vi "TEST_InputDevice.vi"() -> ()   [LabVIEW 2021, in "InputDevice.lvlib"]
uses:
  InputDevice.lvlib
  Joystick/Joystick.lvclass
  Keyboard/Keyboard.lvclass
  Mouse/Mouse.lvclass
  <vilib>/ErrorRing/Error Ring.xnode
  InputDevice.lvclass
  5e27b7e4-08c8-4db0-82d1-7d7273c4f812.vi
  <vilib>/Utility/miscctls.llb/LVPoint32TypeDef.ctl
panel:
  out "mouse info":T1(array[cluster])
  out "key info":T2(array[cluster])
  out "joystick info":T3(array[cluster])
  out "Joystick B Info Button 1":bool
  out "Joystick Axis Events":T4
  out "Joy Direction Event":T5
  out "Keys Pressed":T6(array[ring])
  out "Button Info Event":T7
  out "Mouse Axis Info Event":T8
  out "Coords":T9
  out "Button":u16
  out "Mods":cluster{"Double Click":bool, "Menu Key":bool}
  out "PlatMods":T10
  in  "stop":bool
  # "Pane Mouse Down"
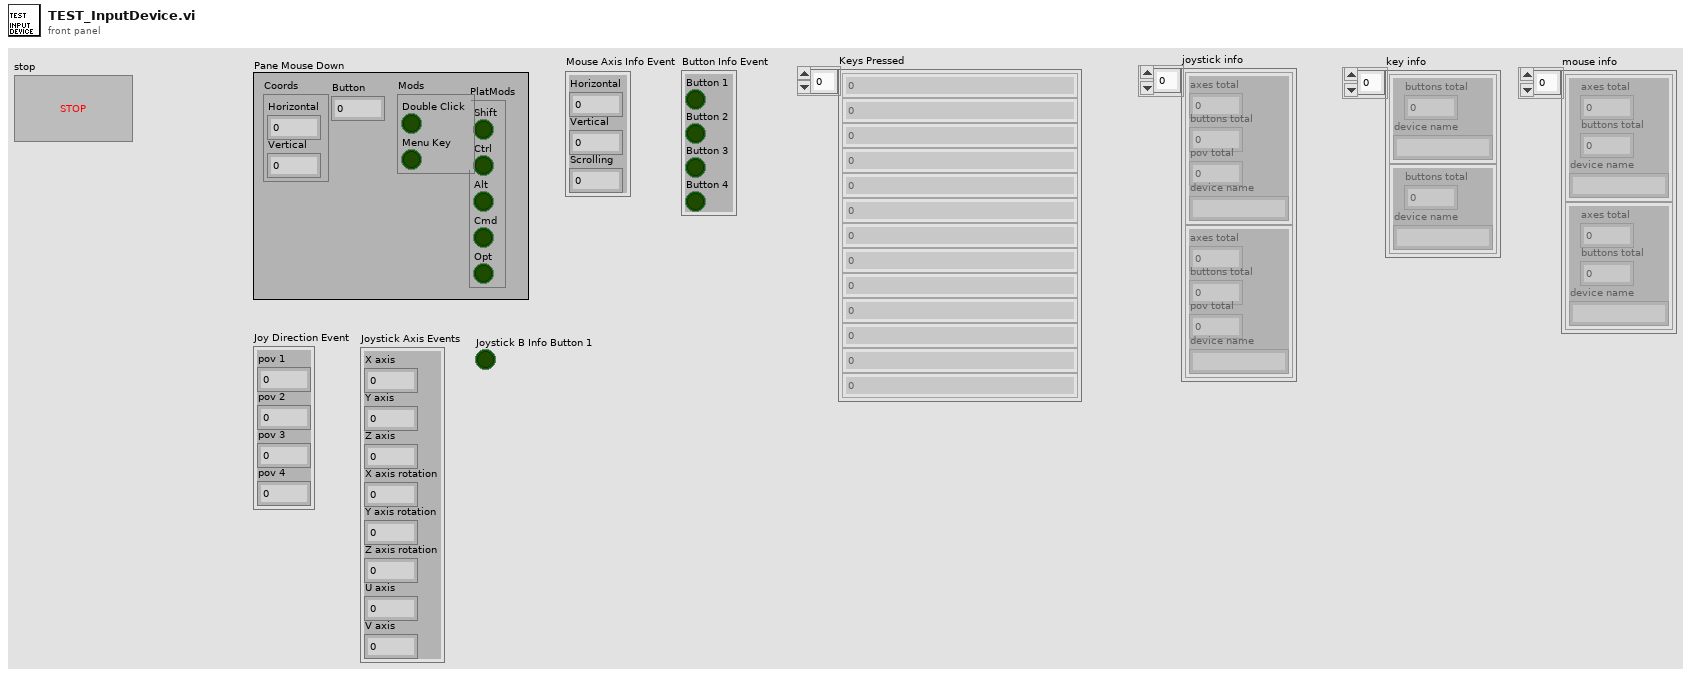
[diagram p1: front panel]
types:
  T1 = cluster{"axes total":u32, "buttons total":u32, "device name":string}[]
  T2 = cluster{"buttons total":u32, "device name":string}[]
  T3 = cluster{"axes total":u32, "buttons total":u32, "pov total":u32, "device name":string}[]
  T4 = cluster{"X axis":i32, "Y axis":i32, "Z axis":i32, "X axis rotation":i32, "Y axis rotation":i32, "Z axis rotation":i32, "U axis":i32, "V axis":i32}
  T5 = cluster{"pov 1":i32, "pov 2":i32, "pov 3":i32, "pov 4":i32}
  T6 = enum16{"0", "1", "2", "3", "4", "5", "6", "7", "8", "9", "A", "B", "C", "D", "E", "F", "G", "H", "I", "J", "K", "L", "M", "N", "O", "P", "Q", "R", "S", "T", "U", "V", "W", "X", "Y", "Z", "F1", "F2", "F3", "F4", "F5", "F6", "F7", "F8", "F9", "F10", "F11", "F12", "F13", "F14", "F15", "ADD", "BACK", "BACKSLASH", "CAPITAL", "COMMA", "DECIMAL", "DELETE", "DIVIDE", "DOWN", "END", "EQUALS", "ESCAPE", "GRAVE (`)", "HOME", "INSERT", "LBRACKET", "LCONTROL", "LEFT", "L ALT", "LSHIFT", "LWIN", "MINUS", "MULTIPLY", "NEXT", "NUMLOCK", "NUMPAD_0", "NUMPAD_1", "NUMPAD_2", "NUMPAD_3", "NUMPAD_4", "NUMPAD_5", "NUMPAD_6", "NUMPAD_7", "NUMPAD_8", "NUMPAD_9", "PAUSE", "PERIOD", "PRIOR (PG UP)", "RBRACKET", "RCONTROL", "RETURN", "RIGHT", "R ALT", "RSHIFT", "RWIN", "SCROLL", "SEMICOLON", "SLASH", "SPACE", "SUBTRACT", "TAB", "UP", "ENTER (num pad)", "' (quote)"}[]
  T7 = cluster{"Button 1":bool, "Button 2":bool, "Button 3":bool, "Button 4":bool}
  T8 = cluster{"Horizontal":i32, "Vertical":i32, "Scrolling":i32}
  T9 = typedef "LVPoint32TypeDef.ctl" = cluster{"Horizontal":i32, "Vertical":i32}
  T10 = cluster{"Shift":bool, "Ctrl":bool, "Alt":bool, "Cmd":bool, "Opt":bool}
  T11 = cluster{"Mouse out":refnum<class "Joystick.lvclass">, "Keyboard out":refnum<class "Keyboard.lvclass">, "Mouse out":refnum<class "Mouse.lvclass">}
  T12 = cluster{"Joystick":refnum<event-registration>, "Keyboard":refnum<event-registration>, "Mouse":refnum<event-registration>}
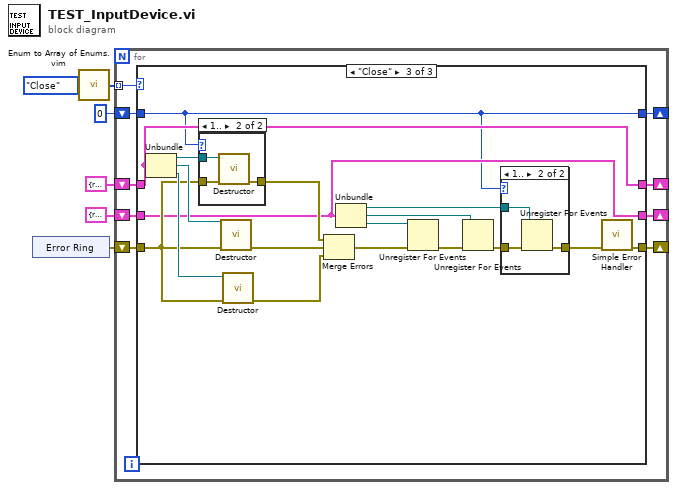
[diagram p0: block diagram]
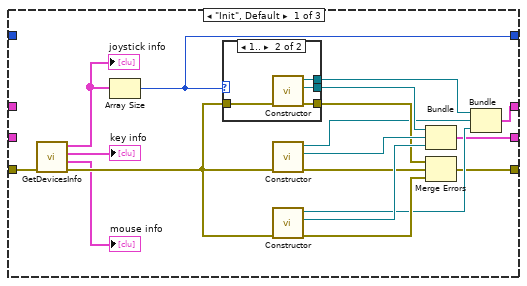
[diagram p2: hidden frame]
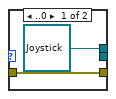
[diagram p3: hidden frame]
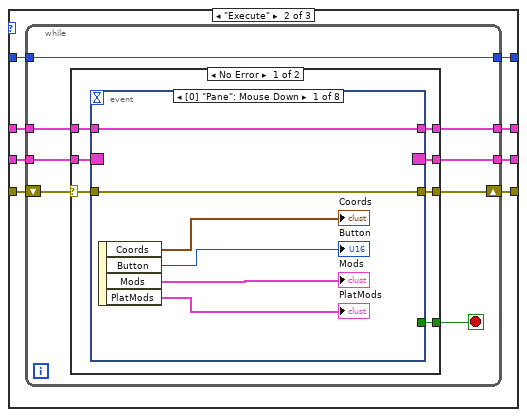
[diagram p4: hidden frame]
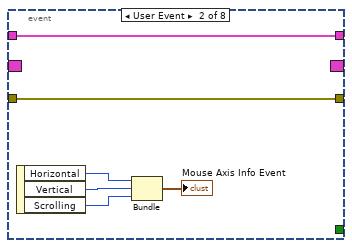
[diagram p5: hidden frame]
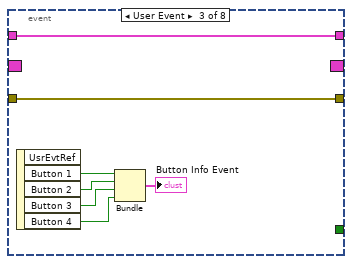
[diagram p6: hidden frame]
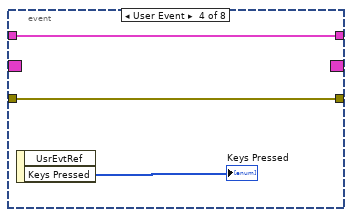
[diagram p7: hidden frame]
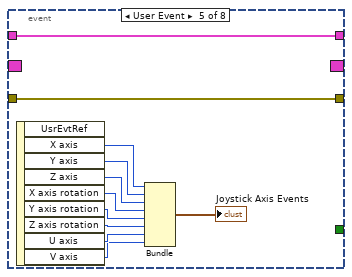
[diagram p8: hidden frame]
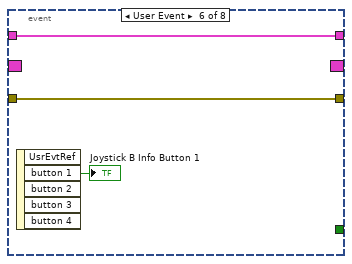
[diagram p9: hidden frame]
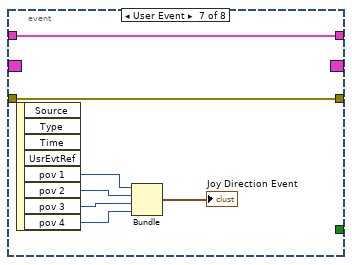
[diagram p10: hidden frame]
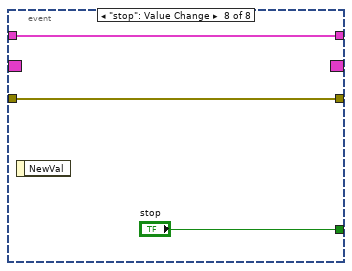
[diagram p11: hidden frame]
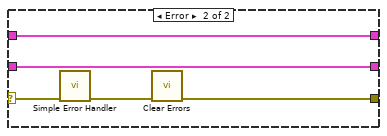
[diagram p12: hidden frame]
diagram:
  n1 = xnode "Error Ring"() -> ("error out"=w3:errorcluster)
  n2 = call "Enum to Array of Enums.vim"("enum"=enum16{"Init", "Execute", "Close"}."Close") -> ("array of enums"=w6:enum16{"Init", "Execute", "Close"}[])
  n3 = for {
    shift-right: [w10] -> _
    shift-left: T12 {"Joystick"=refnum, "Keyboard"=refnum, "Mouse"=refnum} -> [w15]
    shift-right: [w9] -> _
    shift-left: w3 -> [w14]
    tunnel: w6 -> [w13] mode=indexing
    shift-right: [w8] -> _
    shift-left: 0 -> [w11]
    shift-right: [w12] -> _
    shift-left: T11 {"Mouse out"=refnum, "Keyboard out"=refnum, "Mouse out"=refnum} -> [w7]
    n4 = case shown="\"Close\"" w13 {
      tunnel: w15 -> [_ w47 w115]
      tunnel: [w17 w46 w117] -> w9
      tunnel: w14 -> [w16 w45 w120]
      tunnel: [w18 w44 w115] -> w10
      tunnel: [w23 w42 w114] -> w8
      tunnel: [w19 w41 w116] -> w12
      tunnel: w7 -> [_ w40 w116]
      tunnel: w11 -> [_ w43 w114]
      frame "Init", Default {
        n5 = call "GetDevicesInfo.vi"("error in (no error)"=w16) -> ("error out"=w33:errorcluster, "mouse info"=→"mouse info":T1, "key info"=→"key info":T2, "joystick info"=w30:T3)  [unwired: 7 in]
        "joystick info" <- w30
        n6 = Array Size(array=w30) -> (size(s)=w23:i32)
        n7 = case shown="1.." w23 {
          tunnel: [w34 w39] -> w24
          tunnel: [refnum<class "Joystick.lvclass"> refnum ("Mouse out") w38] -> w22
          tunnel: [_ w37] -> w27
          tunnel: w33 -> [w34 w36]
          frame ..0 {
          }
          frame 1.. {
            n8 = call "Constructor.vi"("error in (no error)"=w36) -> ("error out"=w39:errorcluster, "Joystick"=w37:refnum<event-registration>, "Mouse out"=w38:refnum<class "Joystick.lvclass">)  [unwired: 8 in]
          }
        }
        n9 = call "Constructor.vi"("error in (no error)"=w33) -> ("error out"=w25:errorcluster, "Keyboard"=w28:refnum<event-registration>, "Keyboard out"=w21:refnum<class "Keyboard.lvclass">)  [unwired: 8 in]
        n10 = call "Constructor.vi"("error in (no error)"=w33) -> ("error out"=w26:errorcluster, "Mouse"=w29:refnum<event-registration>, "Mouse out"=w20:refnum<class "Mouse.lvclass">)  [unwired: 8 in]
        n11 = Bundle("Joystick"=w27, "Keyboard"=w28, "Mouse"=w29) -> (w18:T12)  [unwired: 1 in]
        n12 = Merge Errors(w24, w25, w26) -> (w17:errorcluster)
        n13 = Bundle("Mouse out"=w22, "Keyboard out"=w21, "Mouse out"=w20) -> (w19:T11)  [unwired: 1 in]
      }
      frame "Execute" {
        n14 = while {
          tunnel: w47 -> [w54]
          tunnel: [w53] -> w44
          shift-right: [w51] -> w46
          shift-left: w45 -> [w52]
          tunnel: [w50] -> w42
          tunnel: w43 -> [w50]
          tunnel: w40 -> [w49]
          tunnel: [w48] -> w41
          stop <- w55 stop-if-true
          n15 = case shown="No Error" w52 {
            selector: w52 -> [w60 w113]
            tunnel: [w62 _] -> w55
            tunnel: w54 -> [w58 w110]
            tunnel: [w61 w110] -> w53
            tunnel: [w59 w111] -> w51
            tunnel: w49 -> [w57 w109]
            tunnel: [w56 w109] -> w48
            frame No Error {
              n16 = event shown="[0] \"Pane\": Mouse Down" {
                selector: w58 -> [_ _ _ _ _ _ _ _]
                dyn-events: [_ _ _ _ _ _ _ _] -> w61
                timeout: _ -> [_ _ _ _ _ _ _ _]
                tunnel: [_ _ _ _ _ _ _ "stop"] -> w62
                tunnel: w60 -> [w64 w70 w76 w84 w95 w98 w105 w107]
                tunnel: [w64 w70 w76 w84 w95 w98 w105 w107] -> w59
                tunnel: w57 -> [w63 w69 w75 w82 w85 w96 w99 w106]
                tunnel: [w63 w69 w75 w82 w85 w96 w99 w106] -> w56
                event Mouse Down {
                  n17 = event-data() -> ("Coords"=→"Coords":T9, "Button"=→"Button":u16, "Mods"=→"Mods":cluster{"Double Click":bool, "Menu Key":bool}, "PlatMods"=→"PlatMods":T10)  [unwired: 1 in]
                }
                event User Event {
                  n18 = event-data() -> ("Horizontal"=w74:i32, "Vertical"=w73:i32, "Scrolling"=w72:i32)  [unwired: 1 in]
                  n19 = Bundle("Horizontal"=w74, "Vertical"=w73, "Scrolling"=w72) -> (→"Mouse Axis Info Event":T8)  [unwired: 1 in]
                }
                event User Event {
                  n20 = event-data() -> ("Button 1"=w81:bool, "Button 2"=w80:bool, "Button 3"=w79:bool, "Button 4"=w78:bool)  [unwired: 1 in, 1 out]
                  n21 = Bundle("Button 1"=w81, "Button 2"=w80, "Button 3"=w79, "Button 4"=w78) -> (→"Button Info Event":T7)  [unwired: 1 in]
                }
                event User Event {
                  n22 = event-data() -> ("Keys Pressed"=→"Keys Pressed":T6)  [unwired: 1 in, 1 out]
                }
                event User Event {
                  n23 = event-data() -> ("X axis"=w94:i32, "Y axis"=w93:i32, "Z axis"=w92:i32, "X axis rotation"=w91:i32, "Y axis rotation"=w90:i32, "Z axis rotation"=w89:i32, "U axis"=w88:i32, "V axis"=w87:i32)  [unwired: 1 in, 1 out]
                  n24 = Bundle("X axis"=w94, "Y axis"=w93, "Z axis"=w92, "X axis rotation"=w91, "Y axis rotation"=w90, "Z axis rotation"=w89, "U axis"=w88, "V axis"=w87) -> (→"Joystick Axis Events":T4)  [unwired: 1 in]
                }
                event User Event {
                  n25 = event-data() -> ("button 1"=→"Joystick B Info Button 1":bool)  [unwired: 1 in, 4 out]
                }
                event User Event {
                  n26 = event-data() -> ("pov 1"=w104:i32, "pov 2"=w103:i32, "pov 3"=w102:i32, "pov 4"=w101:i32)  [unwired: 1 in, 4 out]
                  n27 = Bundle("pov 1"=w104, "pov 2"=w103, "pov 3"=w102, "pov 4"=w101) -> (→"Joy Direction Event":T5)  [unwired: 1 in]
                }
                event "stop": Value Change {
                  n28 = event-data() -> ()  [unwired: 1 in, 1 out]
                }
              }
            }
            frame Error {
              n29 = call <vilib>:"Simple Error Handler.vi"("error in (no error)"=w113) -> ("error out"=w112:errorcluster)  [unwired: 4 in, 4 out]
              n30 = call <vilib>:"Clear Errors.vi"("error in (no error)"=w112) -> ("error out"=w111:errorcluster)  [unwired: 5 in, 1 out]
            }
          }
        }
      }
      frame "Close" {
        n31 = Unbundle(w116) -> ("Mouse out"=w123:refnum<class "Joystick.lvclass">, "Keyboard out"=w122:refnum<class "Keyboard.lvclass">, "Mouse out"=w121:refnum<class "Mouse.lvclass">)
        n32 = case shown="1.." w114 {
          tunnel: [w136 w139] -> w125
          tunnel: w123 -> [_ w138]
          tunnel: w120 -> [w136 w137]
          frame ..0 {
          }
          frame 1.. {
            n33 = call-dynamic "Destructor.vi"("error in (no error)"=w137, "Mouse in"=w138) -> ("error out"=w139:errorcluster)  [unwired: 9 in]
          }
        }
        n34 = call-dynamic "Destructor.vi"("error in (no error)"=w120, "Mouse in"=w122) -> ("error out"=w124:errorcluster)  [unwired: 9 in]
        n35 = call-dynamic "Destructor.vi"("error in (no error)"=w120, "Mouse in"=w121) -> ("error out"=w126:errorcluster)  [unwired: 9 in]
        n36 = Merge Errors(w125, w124, w126) -> (w127:errorcluster)
        n37 = Unbundle(w115) -> ("Joystick"=w131:refnum<event-registration>, "Keyboard"=w119:refnum<event-registration>, "Mouse"=w118:refnum<event-registration>)
        n38 = Unregister For Events(event registration refnum=w118, error in=w127) -> (error out=w128:errorcluster)
        n39 = Unregister For Events(event registration refnum=w119, error in=w128) -> (error out=w129:errorcluster)
        n40 = case shown="1.." w114 {
          tunnel: w129 -> [w132 w135]
          tunnel: [w132 w134] -> w130
          tunnel: w131 -> [_ w133]
          frame ..0 {
          }
          frame 1.. {
            n41 = Unregister For Events(event registration refnum=w133, error in=w135) -> (error out=w134:errorcluster)
          }
        }
        n42 = call <vilib>:"Simple Error Handler.vi"("error in (no error)"=w130) -> ("error out"=w117:errorcluster)  [unwired: 4 in, 4 out]
      }
    }
  }
